vi "Overlay.vi"(8 "error in (no error)":errorcluster, 10 "Image In":T1, 11 "Overlay Base in":refnum<class "Analyze Results Fluence and Energy.lvclass">) -> (0 "error out":errorcluster, 2 "Image out":T1, 3 "Overlay Base out":refnum<class "Analyze Results Fluence and Energy.lvclass">)   [LabVIEW 2014, in "Analyze Results Fluence and Energy.lvclass"]
uses:
  Analyze Results Fluence and Energy.lvclass
  <vilib>/vision/Image Controls.llb/IMAQ Image.ctl
  Analyze Results Fluence and Energy.lvclass/Analyze Results Fluence and Energy.ctl
  JETI200 Overview and ShotID/HIJ Vision/Analyze/Results and Overlays/Results Base/Analyze Results Base.lvclass
  JETI200 Overview and ShotID/HIJ Vision/Analyze/Results and Overlays/Results Energy/Analyze Results Energy.lvclass
  JETI200 Overview and ShotID/HIJ Vision/Analyze/Results and Overlays/Results Fluence/Analyze Results Fluence.lvclass
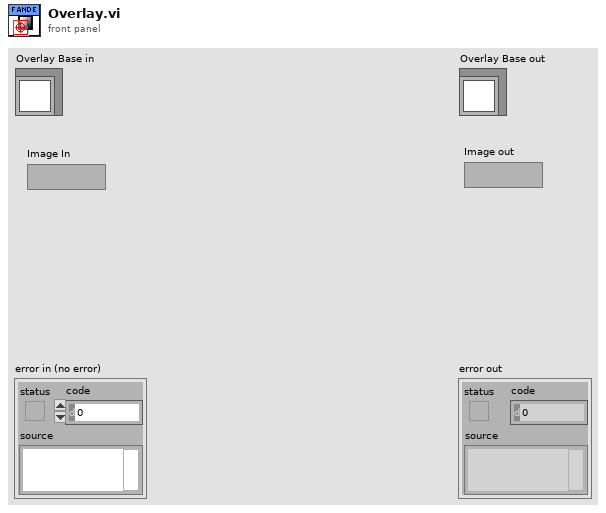
[diagram p1: front panel]
types:
  T1 = typedef "IMAQ Image.ctl" = refnum<image>
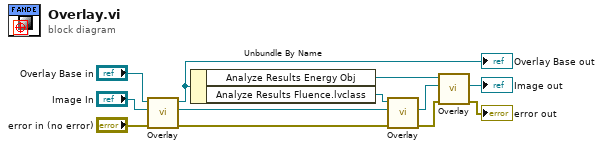
[diagram p0: block diagram]
diagram:
  n1 = call-parent "Overlay.vi"("error in (no error)"="error in (no error)", "Image In"="Image In", "Overlay Base in"="Overlay Base in") -> ("error out"=w2:errorcluster, "Image out"=w5:T1, "Overlay Base out"=w9:refnum<class "Analyze Results Fluence and Energy.lvclass">)  [unwired: 6 in]
  "Overlay Base out" <- w9
  n2 = Unbundle By Name(w9) -> ("Analyze Results Energy Obj"=w8:refnum<class "Analyze Results Energy.lvclass">, "Analyze Results Fluence.lvclass"=w6:refnum<class "Analyze Results Fluence.lvclass">)
  n3 = call-dynamic "Overlay.vi"("error in (no error)"=w2, "Image In"=w5, "Overlay Base in"=w6) -> ("error out"=w7:errorcluster, "Image out"=w4:T1)  [unwired: 6 in, 1 out]
  n4 = call-dynamic "Overlay.vi"("error in (no error)"=w7, "Image In"=w4, "Overlay Base in"=w8) -> ("error out"=→"error out":errorcluster, "Image out"=→"Image out":T1)  [unwired: 6 in, 1 out]
